vi "UDP Configuration Test.vi"() -> ()   [LabVIEW 2016]
uses:
  Source/Shared/Typedefs/DSF.Shared.Typedefs.Configuration.Transfer.Channel Descriptor.ctl
  Source/Shared/Typedefs/DSF.Shared.Typedefs.Configuration.Transfer.Channel Parameters.ctl
  Source/Shared/Typedefs/DSF.Shared.Typedefs.Data Type.ctl
  <vilib>/NI Veristand/Custom Device API/Custom Device Item Ref.ctl
  Source/Shared/Typedefs/DSF.Shared.Typedefs.Direction.ctl
  Source/Shared/Typedefs/DSF.Shared.Typedefs.Cycle Timing Factors.ctl
  UDP/DSF.UDP.Configuration.Plugin.lvclass
  C:/Git/SourceTree/DSF/Source/Shared/Classes/Configuration/DSF.Shared.Configuration.lvclass
  C:/Git/SourceTree/DSF/Source/Shared/Classes/Plugin/DSF.Shared.Configuration.Plugin.lvclass
  Source/Shared/Classes/Plugin/DSF.Shared.Configuration.Plugin.lvclass/DSF.Shared.Configuration.Plugin.ctl
  Source/Shared/Classes/Transfer Group/DSF.Shared.Configuration.Transfer Group.lvclass/DSF.Shared.Configuration.Transfer Group.ctl
  Source/Shared/Classes/Transfer/DSF.Shared.Configuration.Transfer.lvclass/DSF.Shared.Configuration.Transfer.ctl
  Source/Shared/Classes/Configuration/DSF.Shared.Configuration.lvclass/DSF.Shared.Configuration.ctl
  Source/Shared/Classes/Transfer Group/DSF.Shared.Configuration.Transfer Group.lvclass
  Source/Shared/Classes/Transfer/DSF.Shared.Configuration.Transfer.lvclass
  UDP/DSF.UDP.Configuration.Transfer.lvclass
  UDP/DSF.UDP.Configuration.Transfer Group.lvclass
  Source/DSF.Shared.lvlib
  Source/Shared/Classes/Configuration/DSF.Shared.Configuration.lvclass
  Source/Shared/Classes/Plugin/DSF.Shared.Configuration.Plugin.lvclass
  <vilib>/NI Veristand/Custom Device API/Custom Device API.lvlib
panel:
  out "Channel Descriptors":T1[](array[typedef]) {"VS Channel Ref" format="%016x"; "Channel Parameters"."offset" format="%d bytes"}
  out "transfer name":string
  out "group name":string
  in  "Direction":T5
  in  "IP Address":string="localhost"
  in  "Port":u16=5000
  in  "Channel Descriptors":T1[](array[typedef])=[{"Channel Parameters"={"offset"=0, "data type"=enum."DBL"}, "VS Channel Ref"=0}, {"Channel Parameters"={"offset"=8, "data type"=enum."DBL"}, "VS Channel Ref"=8}, {"Channel Parameters"={"offset"=16, "data type"=enum."Bool"}, "VS Channel Ref"=16}] {"VS Channel Ref" format="%016x"; "Channel Parameters"."offset" format="%d bytes"}
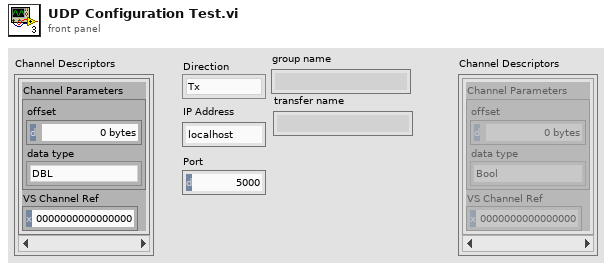
[diagram p1: front panel]
types:
  T1 = typedef "DSF.Shared.lvlib/DSF.Shared.Typedefs.Configuration.Transfer.Channel Descriptor.ctl" = cluster{"Channel Parameters":T2, "VS Channel Ref":T4}
  T2 = typedef "DSF.Shared.lvlib/DSF.Shared.Typedefs.Configuration.Transfer.Channel Parameters.ctl" = cluster{"offset":u64, "data type":T3}
  T3 = typedef "DSF.Shared.lvlib/DSF.Shared.Typedefs.Data Type.ctl" = enum8{"Bool", "SGL", "DBL", "I8", "I16", "I32", "I64", "U8", "U16", "U32", "U64"}
  T4 = typedef "Custom Device API.lvlib/Custom Device Item Ref.ctl" = u64
  T5 = typedef "DSF.Shared.lvlib/DSF.Shared.Typedefs.Direction.ctl" = enum16{"Tx", "Rx"}
  T6 = typedef "DSF.Shared.lvlib/DSF.Shared.Typedefs.Cycle Timing Factors.ctl" = cluster{"Decimation":u64, "Offset":u64}
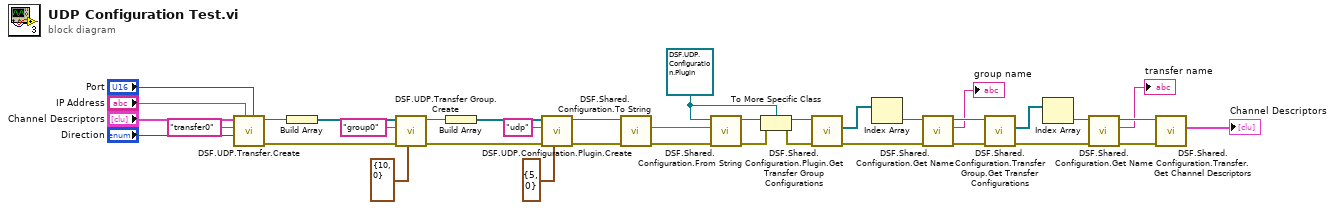
[diagram p0: block diagram]
diagram:
  w14 = refnum<class "DSF.UDP.Configuration.Plugin.lvclass"> refnum ("UDP Plugin Configuration out")
  n1 = call "DSF.UDP.Transfer.Create.vi"("Port"="Port", "IP Address"="IP Address", "Direction"="Direction", "Name"="transfer0", "Channel Descriptors"="Channel Descriptors") -> ("error out"=w34:errorcluster, "UDP Transfer out"=w36:refnum<class "DSF.UDP.Configuration.Transfer.lvclass">)  [unwired: 5 in]
  n2 = Build Array(w36) -> (w35:refnum<class "DSF.UDP.Configuration.Transfer.lvclass">[])
  n3 = call "DSF.UDP.Transfer Group.Create.vi"("Cycle Timing Factors"=T6 {"Decimation"=10, "Offset"=0}, "error in (no error)"=w34, "Name"="group0", "UDP Transfer Configurations"=w35) -> ("error out"=w25:errorcluster, "UDP Transfer Group out"=w27:refnum<class "DSF.UDP.Configuration.Transfer Group.lvclass">)  [unwired: 6 in]
  n4 = Build Array(w27) -> (w26:refnum<class "DSF.UDP.Configuration.Transfer Group.lvclass">[])
  n5 = call "DSF.UDP.Configuration.Plugin.Create.vi"("Cycle Timing Factors"=T6 {"Decimation"=5, "Offset"=0}, "error in (no error)"=w25, "Name"="udp", "UDP Transfer Group Configurations"=w26) -> ("error out"=w21:errorcluster, "UDP Plugin Configuration out"=w22:refnum<class "DSF.UDP.Configuration.Plugin.lvclass">)  [unwired: 6 in]
  n6 = call "DSF.Shared.Configuration.To String.vi"("error in (no error)"=w21, "Configuration in"=w22) -> ("error out"=w19:errorcluster, "String"=w20:string)  [unwired: 7 in, 1 out]
  n7 = call "DSF.Shared.Configuration.From String.vi"("error in (no error)"=w19, "String"=w20, "Configuration in"=w14) -> ("error out"=w17:errorcluster, "Configuration out"=w16:refnum<class "DSF.Shared.Configuration.lvclass">)  [unwired: 7 in]
  n8 = To More Specific Class(target class=w14, reference=w16, error in=w17) -> (specific class reference=w15:refnum<class "DSF.UDP.Configuration.Plugin.lvclass">, error out=w18:errorcluster)
  n9 = call "DSF.Shared.Configuration.Plugin.Get Transfer Group Configurations.vi"("error in (no error)"=w18, "Plugin Configuration in"=w15) -> ("error out"=w12:errorcluster, "Transfer Group Configurations"=w13:refnum<class "DSF.Shared.Configuration.Transfer Group.lvclass">[])  [unwired: 7 in, 1 out]
  n10 = Index Array(array=w13) -> (element=w11:refnum<class "DSF.Shared.Configuration.Transfer Group.lvclass">)  [unwired: 1 in]
  n11 = call "DSF.Shared.Configuration.Get Name.vi"("error in (no error)"=w12, "Configuration in"=w11) -> ("error out"=w10:errorcluster, "Name"=→"group name":string, "Configuration out"=w9:refnum<class "DSF.Shared.Configuration.Transfer Group.lvclass">)  [unwired: 7 in]
  n12 = call "DSF.Shared.Configuration.Transfer Group.Get Transfer Configurations.vi"("error in (no error)"=w10, "Transfer Group Configuration in"=w9) -> ("error out"=w6:errorcluster, "Transfer Configurations"=w7:refnum<class "DSF.Shared.Configuration.Transfer.lvclass">[])  [unwired: 7 in, 1 out]
  n13 = Index Array(array=w7) -> (element=w5:refnum<class "DSF.Shared.Configuration.Transfer.lvclass">)  [unwired: 1 in]
  n14 = call "DSF.Shared.Configuration.Get Name.vi"("error in (no error)"=w6, "Configuration in"=w5) -> ("error out"=w4:errorcluster, "Name"=→"transfer name":string, "Configuration out"=w3:refnum<class "DSF.Shared.Configuration.Transfer.lvclass">)  [unwired: 7 in]
  n15 = call "DSF.Shared.Configuration.Transfer.Get Channel Descriptors.vi"("error in (no error)"=w4, "Transfer Configuration in"=w3) -> ("Channel Descriptors"=→"Channel Descriptors":T1[])  [unwired: 7 in, 2 out]
